vi "Find all IFD locations from file.vi"(8 "error in":errorcluster, 11 "File":refnum<file>) -> (0 "error out":errorcluster, 1 "Location in byte stream of\n Long Word that points to the last IFD.\n\nThis is the Word to change if you are adding another page\nto the file.":u32, 2 "IFD locations":u32[](array[numeric]), 3 "File":refnum<file>, 4 "1st tag locations":u32[](array[numeric]), 5 "# of tags in each IFD":u16[](array[numeric]), 7 "Litt/BigEnd":bool)   [LabVIEW 2013, in "Tiff reader.lvlib"]
doc: "Read all IFD location via reading directly from the file."
uses:
  Tiff reader.lvlib
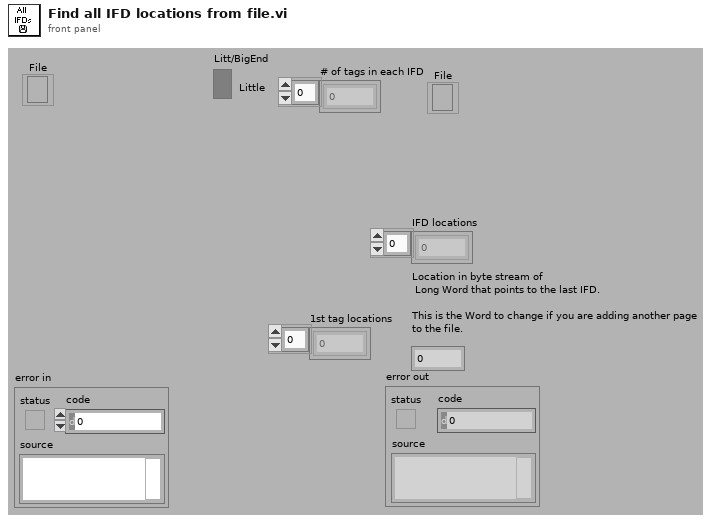
[diagram p1: front panel]
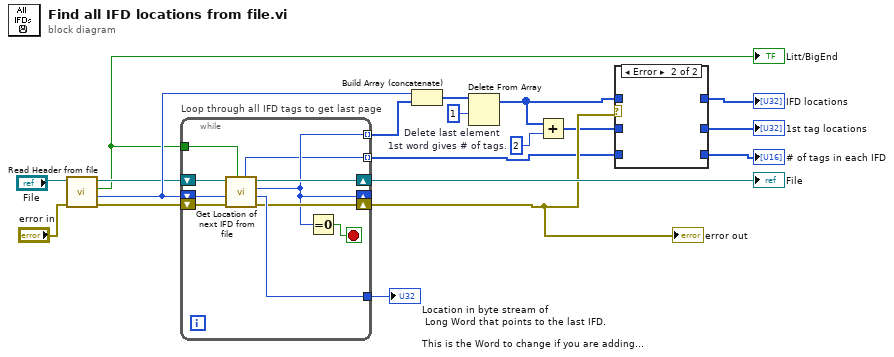
[diagram p0: block diagram]
diagram:
  w8 = u32 2  # 1st word gives # of tags.
  n1 = call "Read Header from file.vi"("error in"="error in", "File"="File") -> ("error out"=w10:errorcluster, "ImFileDirectOffs"=w14:u32, "Litt/BigEnd"=w11:bool, "File"=w13:refnum<file>)  [unwired: 4 out]
  "Litt/BigEnd" <- w11
  n2 = while "Loop through all IFD tags to get last page" {
    shift-right: [w21] -> _
    shift-left: w14 -> [w23]
    tunnel: [w25] -> w19
    tunnel: [w21] -> w18 mode=indexing
    shift-right: [w22] -> w12
    shift-left: w13 -> [w28]
    tunnel: w11 -> [w27]
    shift-right: [w24] -> w7
    shift-left: w10 -> [w26]
    tunnel: [w20] -> w1 mode=indexing
    stop <- w29 stop-if-true
    n3 = call "Get Location of next IFD from file.vi"("Litt/BigEnd"=w27, "error in"=w26, "Start of current IFD\n(ImFileDirectOffs)"=w23, "File"=w28) -> ("error out"=w24:errorcluster, "Location in byte stream of \nLong Word that points to this next IFD"=w25:u32, "Location in byte stream of \nnext IFD if there is a next IFD,\n0 otherwise"=w21:u32, "File out"=w22:refnum<file>, "# of tags"=w20:u16)  [unwired: 1 out]
    n4 = Equal To 0?(x=w21) -> (x = 0?=w29:bool)
  }
  "Location in byte stream of\n Long Word that points to the last IFD.\n\nThis is the Word to change if you are adding another page\nto the file." <- w19
  "File" <- w12
  "error out" <- w7
  n5 = Build Array (concatenate)(w14, w18) -> (w17:u32[])
  n6 = Delete From Array "Delete last element"(array=w17, length=1) -> (array with subset deleted=w4:u32[])  [unwired: 1 in, 1 out]
  n7 = Add(x=w4, y=w8) -> (x+y=w5:u32[])
  n8 = case shown="Error" w7 {
    tunnel: [w32 _] -> w6
    tunnel: w5 -> [w32 _]
    tunnel: [w31 _] -> w3
    tunnel: w4 -> [w31 _]
    tunnel: [w30 _] -> w2
    tunnel: w1 -> [w30 _]
    frame No Error {
    }
    frame Error {
    }
  }
  "IFD locations" <- w3
  "# of tags in each IFD" <- w2
  "1st tag locations" <- w6
